vi "EnumTest.vi"() -> ()   [LabVIEW 2014]
panel:
  out "Numeric":dbl
  in  "A":enum16{"a", "b", "c"}(ring)
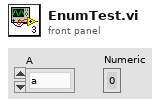
[diagram p1: front panel]
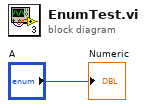
[diagram p0: block diagram]
diagram:
  "Numeric" <- "A"
